vi "PH_4_Pos_Selector.get 6P 4Q Position DIM Service.vi"(1 "no link":bool, 2 "typeDescriptor":string, 3 "data":i8[](array[numeric])) -> (0 "Position":T1 items=["unknown", "Position I", "Position II", "Position III", "Position IV", "moving"])   [LabVIEW 2014, in "PH_4_Pos_Selector.lvlib"]
doc: "This VI calculates the status Sixpack 4 Position tags."
uses:
  PH_4_Pos_Selector.Position Selector.ctl
  PH_4_Pos_Selector.lvlib
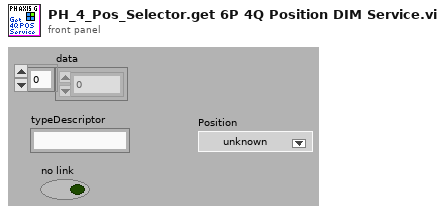
[diagram p1: front panel]
types:
  T1 = typedef "PH_4_Pos_Selector.lvlib/PH_4_Pos_Selector.Position Selector.ctl" = u16
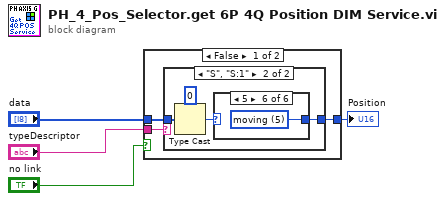
[diagram p0: block diagram]
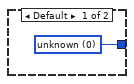
[diagram p2: hidden frame]
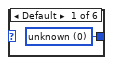
[diagram p3: hidden frame]
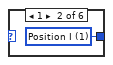
[diagram p4: hidden frame]
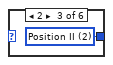
[diagram p5: hidden frame]
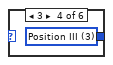
[diagram p6: hidden frame]
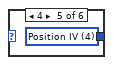
[diagram p7: hidden frame]
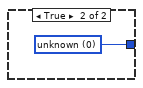
[diagram p8: hidden frame]
diagram:
  n1 = case "No link?" shown="False" "no link" {
    tunnel: [w7 w19] -> w4
    tunnel: "data" -> [w6 _]
    tunnel: "typeDescriptor" -> [w5 _]
    frame False {
      n2 = case "Check data type" shown="\"S\", \"S:1\"" w5 {
        tunnel: [w8 w11] -> w7
        tunnel: w6 -> [_ w9]
        frame Default {
          w8 = T1 0 items=["unknown", "Position I", "Position II", "Position III", "Position IV", "moving"] ("Selector")
        }
        frame "S", "S:1" {
          n3 = Type Cast(type=i16 0, x=w9) -> (*(type *) &x=w10:i16)
          n4 = case shown="5" w10 {
            tunnel: [w13 w14 w15 w16 w17 w18] -> w11
            frame Default {
              w13 = T1 0 items=["unknown", "Position I", "Position II", "Position III", "Position IV", "moving"] ("Selector")
            }
            frame 1 {
              w14 = T1 1 items=["unknown", "Position I", "Position II", "Position III", "Position IV", "moving"] ("Selector")
            }
            frame 2 {
              w15 = T1 2 items=["unknown", "Position I", "Position II", "Position III", "Position IV", "moving"] ("Selector")
            }
            frame 3 {
              w16 = T1 3 items=["unknown", "Position I", "Position II", "Position III", "Position IV", "moving"] ("Selector")
            }
            frame 4 {
              w17 = T1 4 items=["unknown", "Position I", "Position II", "Position III", "Position IV", "moving"] ("Selector")
            }
            frame 5 {
              w18 = T1 5 items=["unknown", "Position I", "Position II", "Position III", "Position IV", "moving"] ("Selector")
            }
          }
        }
      }
    }
    frame True {
      w19 = T1 0 items=["unknown", "Position I", "Position II", "Position III", "Position IV", "moving"] ("Selector")
    }
  }
  "Position" <- w4
